vi "op_biti_v6_01.vi"() -> ()   [LabVIEW 2010]
panel:
  out "Numeric":dbl=181.0
  in  "Array 2":bool[](array[boolean])=[TRUE, FALSE, TRUE, TRUE, FALSE, TRUE, FALSE, TRUE]
  out "Array":bool[](array[boolean])=[TRUE, FALSE, TRUE, TRUE, FALSE, TRUE, FALSE, TRUE]
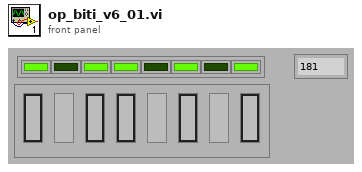
[diagram p1: front panel]
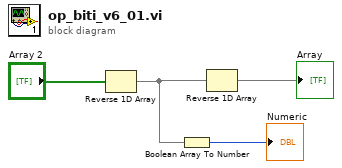
[diagram p0: block diagram]
diagram:
  n1 = Reverse 1D Array(array="Array 2") -> (reversed array=w2:bool[])
  n2 = Boolean Array To Number(Boolean array=w2) -> (number=→"Numeric":u32)
  n3 = Reverse 1D Array(array=w2) -> (reversed array=→"Array":bool[])
